vi "JSON-RPC Errors.vi"(10 "error in":errorcluster, 11 "Enum":T1(ring)) -> (2 "error out":errorcluster)   [LabVIEW 2019, in "JSON-RPC.lvclass"]
uses:
  JSON-RPC.lvclass
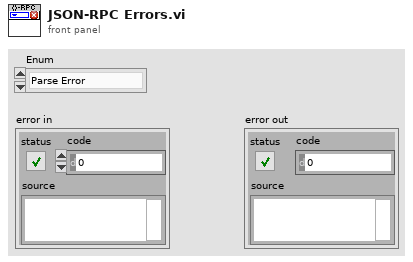
[diagram p1: front panel]
types:
  T1 = enum16{"Parse Error", "Invalid Request", "Method not found", "Invalid params", "Internal error", "Server error"}
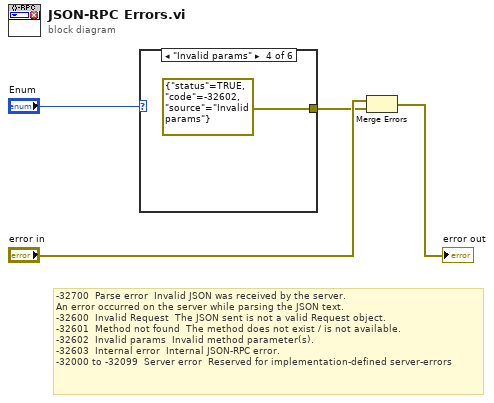
[diagram p0: block diagram]
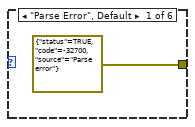
[diagram p2: hidden frame]
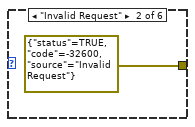
[diagram p3: hidden frame]
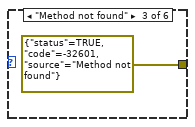
[diagram p4: hidden frame]
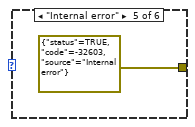
[diagram p5: hidden frame]
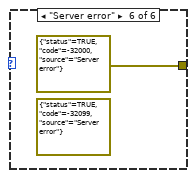
[diagram p6: hidden frame]
diagram:
  # "-32700 \tParse error \tInvalid JSON was received by the server.\nAn error occurred on the server while parsing the JSON text.\n-32600 \tInvalid Request \tThe JSON sent is not a valid Request object.\n-32601 \tMethod not found \tThe method does not exist / is not available.\n-32602 \tInvalid params \tInvalid method parameter(s).\n-32603 \tInternal error \tInternal JSON-RPC error.\n-32000 to -32099 \tServer error \tReserved for implementation-defined server-errors"
  n1 = case shown="\"Invalid params\"" "Enum" {
    tunnel: [errorcluster {"status"=TRUE, "code"=-32700, "source"="Parse error"} ("error out") errorcluster {"status"=TRUE, "code"=-32600, "source"="Invalid Request"} ("error out") errorcluster {"status"=TRUE, "code"=-32601, "source"="Method not found"} ("error out") errorcluster {"status"=TRUE, "code"=-32602, "source"="Invalid params"} ("error out") errorcluster {"status"=TRUE, "code"=-32603, "source"="Internal error"} ("error out") errorcluster {"status"=TRUE, "code"=-32000, "source"="Server error"} ("error out")] -> w2
    frame "Parse Error", Default {
    }
    frame "Invalid Request" {
    }
    frame "Method not found" {
    }
    frame "Invalid params" {
    }
    frame "Internal error" {
    }
    frame "Server error" {
      (unwired) errorcluster {"status"=TRUE, "code"=-32099, "source"="Server error"} ("error out")
    }
  }
  n2 = Merge Errors("error in", w2) -> (→"error out":errorcluster)
